vi "Teleop.vi"(10 "Match Info":T1={"Autonomous Elapsed Seconds"=0.0, "TeleOp Elapsed Seconds"=0.0, "Disabled Elapsed Seconds"=0.0, "Visited Autonomous"=FALSE, "Visited TeleOp"=FALSE, "Visited Disabled"=FALSE, "Autonomous Settings"={"Autonomous Style"=enum."Independent", "VI Refnum"=refnum}}, 11 "Call Context":T2) -> ()   [LabVIEW 2016]
doc: "This VI is called for each TeleOp packet received from the DS where the robot is not disabled. It is often used to read from the joysticks and update I/O or to update setpoints for timed control loops. It should complete and return within 20 milliseconds or it may miss DS packets."
uses:
  <vilib>/Rock Robotics/WPI/DriverStation/WPI_DriverStationDerivedRobotMode.ctl
  <vilib>/Rock Robotics/WPI/DriverStation/WPI_DriverStationMatch Info.ctl
  <vilib>/Rock Robotics/Network Tables/NT Read Boolean.vi
  <vilib>/Rock Robotics/Network Tables/NT Read Number.vi
  <vilib>/Rock Robotics/WPI/Utilities/WPI_GetSetVariantRefNum.vi
  <vilib>/Rock Robotics/Network Tables/NT Write Numeric Array.vi
  <vilib>/Rock Robotics/Network Tables/NT Write Boolean Array.vi
panel:
  out "Lift Bottom":dbl
  out "Lift Top":dbl
  out "Sample Slider 0":dbl(slide) scale=0.0..5.0
  out "Sample Boolean 1":bool
  out "Sample Boolean 0":bool
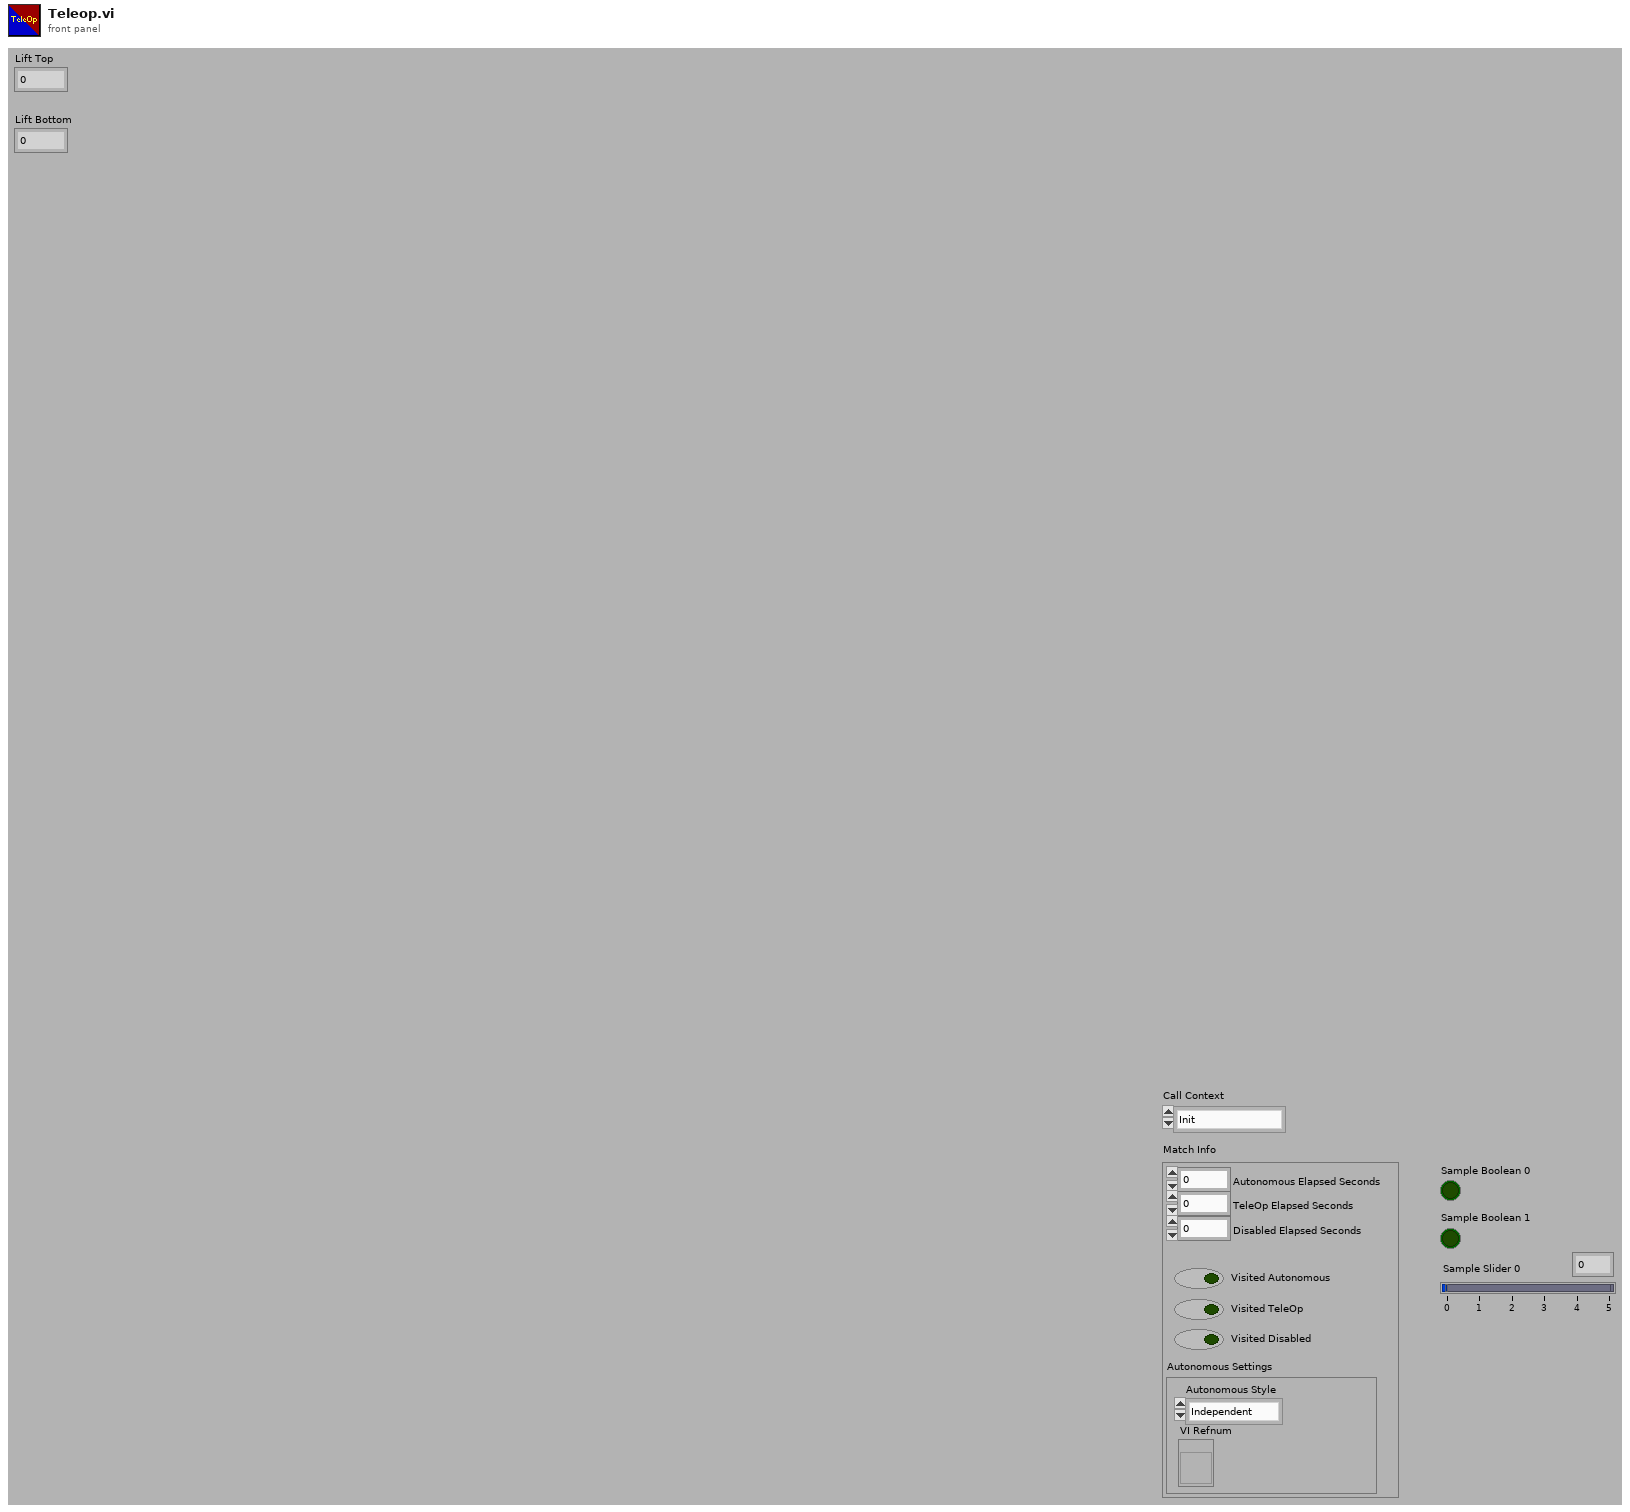
[diagram p1: front panel]
types:
  T1 = typedef "WPI_DriverStationMatch Info.ctl" = cluster{"Autonomous Elapsed Seconds":dbl, "TeleOp Elapsed Seconds":dbl, "Disabled Elapsed Seconds":dbl, "Visited Autonomous":bool, "Visited TeleOp":bool, "Visited Disabled":bool, "Autonomous Settings":cluster{"Autonomous Style":enum16{"Iterative", "Independent"}, "VI Refnum":refnum<vi>}}
  T2 = typedef "WPI_DriverStationDerivedRobotMode.ctl" = enum16{"Init", "Execute", "Stop"}
  T3 = typedef "WPI_JoystickDevRef.ctl" = cluster{"Device":T4}
  T4 = typedef "WPI_JoystickDeviceEnum.ctl" = enum16{"USB 0", "USB 1", "USB 2", "USB 3", "USB 4", "USB 5"}
  T5 = cluster{"Buttons[0]":bool, "Buttons[1]":bool, "Buttons[2]":bool, "Buttons[3]":bool, "Buttons[4]":bool, "Buttons[5]":bool, "Buttons[6]":bool, "Buttons[7]":bool, "Buttons[8]":bool}
  T6 = typedef "WPI_DigitalInputDevRef.ctl" = cluster{"DevStatus":errorcluster, "DIO Channel":T7}
  T7 = typedef "FPGA_DIOChannel.ctl" = enum8{"DIO 0", "DIO 1", "DIO 2", "DIO 3", "DIO 4", "DIO 5", "DIO 6", "DIO 7", "DIO 8", "DIO 9", "DIO MXP 0", "DIO MXP 1", "DIO MXP 2", "DIO MXP 3", "DIO MXP 4", "DIO MXP 5", "DIO MXP 6", "DIO MXP 7", "DIO MXP 8", "DIO MXP 9", "DIO MXP 10", "DIO MXP 11", "DIO MXP 12", "DIO MXP 13", "DIO MXP 14", "DIO MXP 15", "SPI Port CS1", "SPI Port CS2", "SPI Port CS3", "SPI Port MISO", "SPI Port MOSI", "Invalid"}
  T8 = typedef "WPI_RobotDriveDevRef.ctl" = cluster{"DevStatus":errorcluster, "Motors[]":T9[], "Square Inputs":bool, "Max Output":dbl}
  T9 = typedef "WPI_MotorControlDeviceRef.ctl" = cluster{"DeviceStatus":errorcluster, "Type":T10, "PWM":cluster{"PWM Channel":T11, "DeadBand":T12}, "CAN":cluster{"Device Number":u8, "SetOutput VI Ref":variant, "GetOutput VI Ref":variant, "Enable VI Ref":variant, "Disable VI Ref":variant, "Data":variant}, "Invert":bool}
  T10 = typedef "WPI_MotorControlType.ctl" = enum16{"PWM", "CAN"}
  T11 = typedef "FPGA_DIOPWMChannel.ctl" = enum8{"PWM 0", "PWM 1", "PWM 2", "PWM 3", "PWM 4", "PWM 5", "PWM 6", "PWM 7", "PWM 8", "PWM 9", "PWM MXP 0", "PWM MXP 1", "PWM MXP 2", "PWM MXP 3", "PWM MXP 4", "PWM MXP 5", "PWM MXP 6", "PWM MXP 7", "PWM MXP 8", "PWM MXP 9", "Invalid"}
  T12 = typedef "WPI_PWMDeadband.ctl" = cluster{"Name":string, "maxPositivePwm":i32, "minPositivePwm":i32, "centerPwm":i32, "maxNegativePwm":i32, "minNegativePwm":i32, "angularRange":u16}
  T13 = cluster{"Axes[0]":dbl, "Axes[1]":dbl, "Axes[2]":dbl, "Axes[3]":dbl, "Axes[4]":dbl, "Axes[5]":dbl, "Axes[6]":dbl, "Axes[7]":dbl, "Axes[8]":dbl}
  T14 = typedef "WPI_ServoDeviceRef.ctl" = cluster{"DeviceStatus":errorcluster, "PWM Channel":T11, "DeadBand":T12}
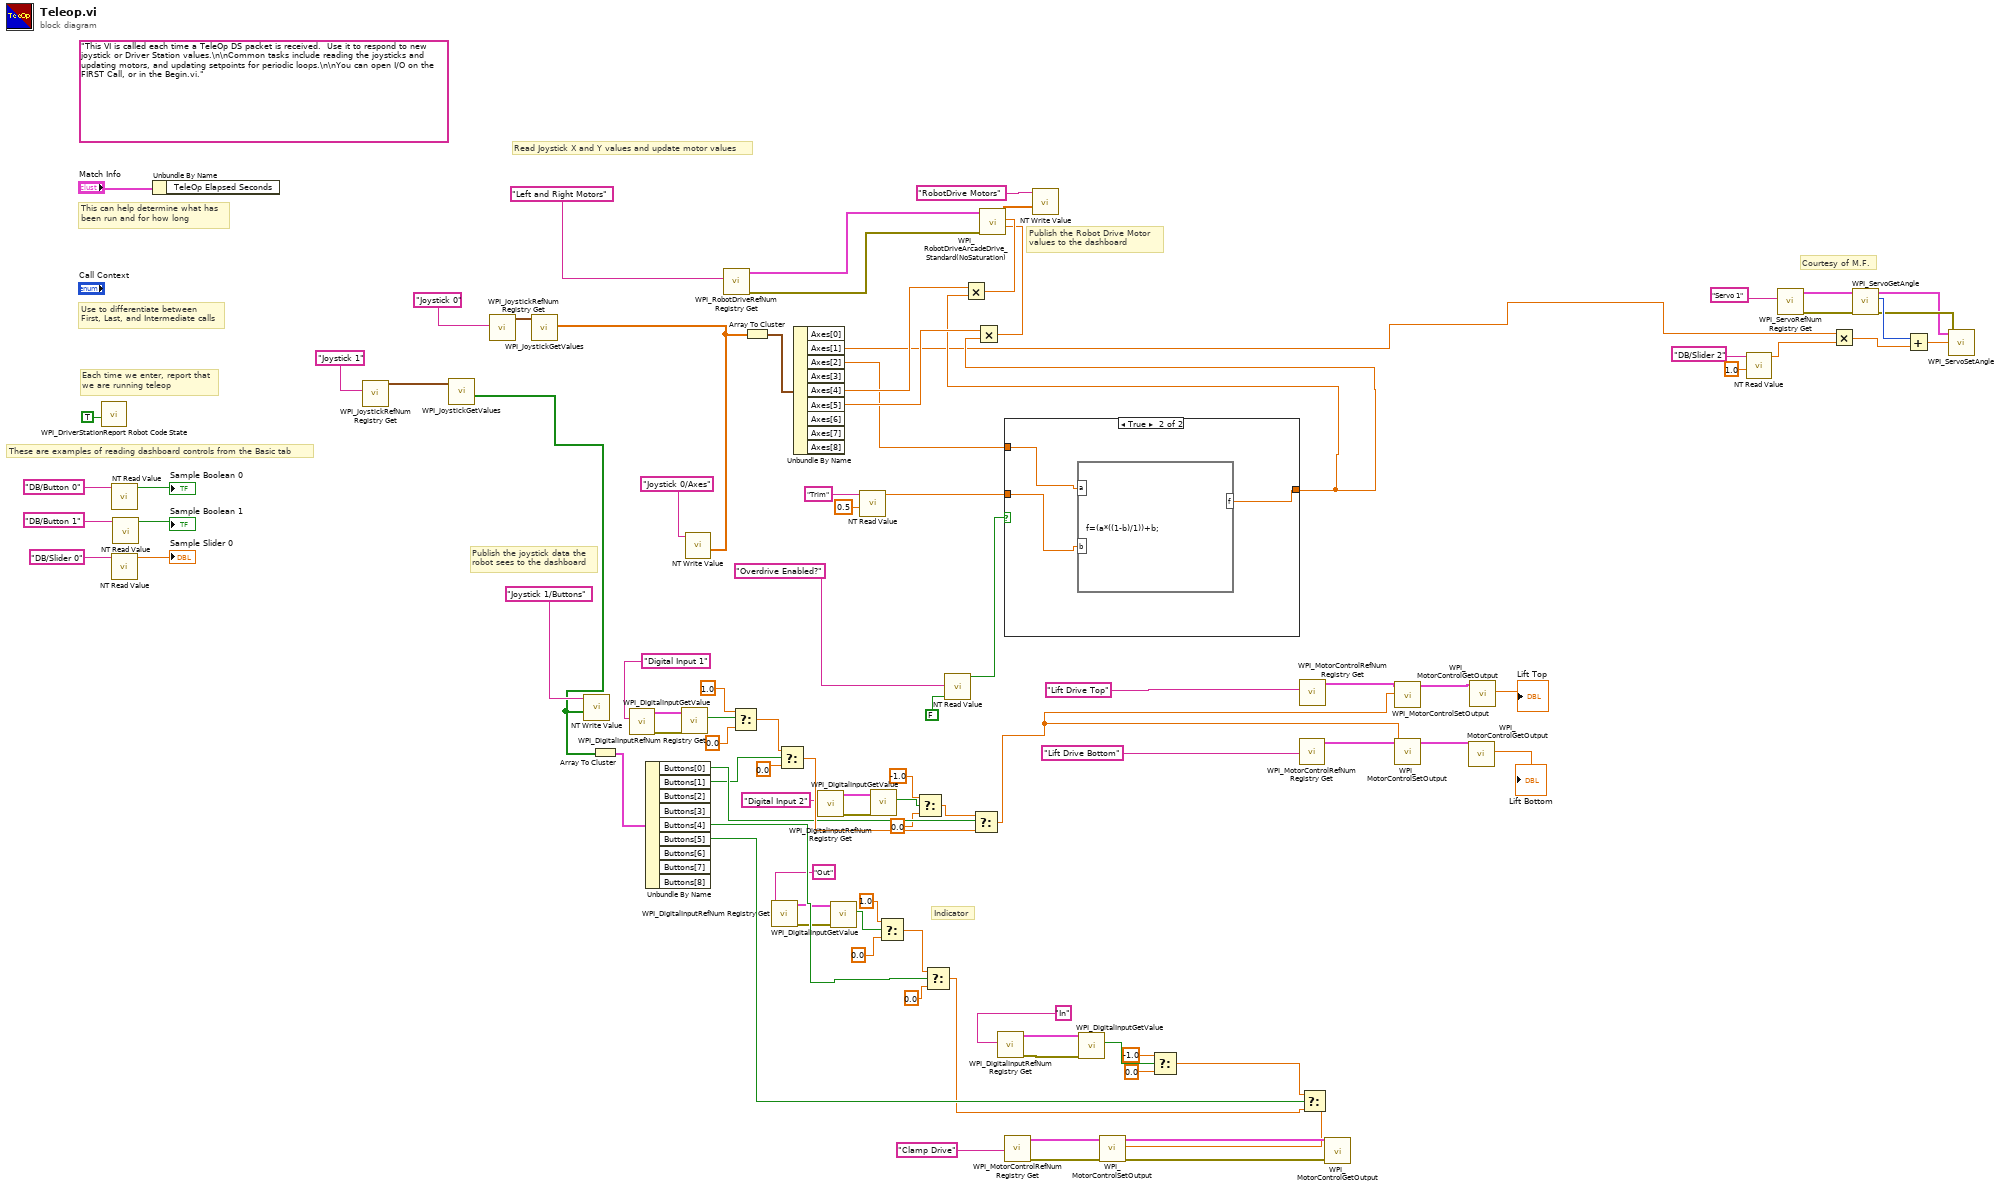
[diagram p0: block diagram]
diagram:
  (unwired) "This VI is called each time a TeleOp DS packet is received.  Use it to respond to new joystick or Driver Station values.\n\nCommon tasks include reading the joysticks and updating motors, and updating setpoints for periodic loops.\n\nYou can open I/O on the FIRST Call, or in the Begin.vi."
  # "Courtesy of M.F."
  # "Indicator"
  # "Publish the Robot Drive Motor\nvalues to the dashboard"
  # "Publish the joystick data the\nrobot sees to the dashboard"
  # "Read Joystick X and Y values and update motor values"
  # "These are examples of reading dashboard controls from the Basic tab"
  # "Each time we enter, report that\nwe are running teleop"
  # "Use to differentiate between\nFirst, Last, and Intermediate calls"
  # "This can help determine what has\nbeen run and for how long"
  n1 = call <vilib>:"WPI_DriverStationReport Robot Code State.vi"("TeleOp"=TRUE ("Autonomous")) -> ()  [unwired: 10 in, 1 out]
  n2 = call-poly <vilib>:"NT Read Value.vi"("Name"="DB/Button 0" ("refnum name")) -> ("Boolean"=→"Sample Boolean 0":bool)  [unwired: 9 in, 1 out]
  n3 = call-poly <vilib>:"NT Read Value.vi"("Name"="DB/Slider 0" ("refnum name")) -> ("Numeric"=→"Sample Slider 0":dbl)  [unwired: 9 in, 1 out]
  n4 = call-poly <vilib>:"NT Read Value.vi"("Name"="DB/Button 1" ("refnum name")) -> ("Boolean"=→"Sample Boolean 1":bool)  [unwired: 9 in, 1 out]
  n5 = Unbundle By Name("Match Info") -> ()  [unwired: 1 out]
  n6 = call <vilib>:"WPI_JoystickRefNum Registry Get.vi"("refnum name"="Joystick 1") -> ("JoystickDevRef"=w49:T3)  [unwired: 9 in, 1 out]
  n7 = call <vilib>:"WPI_JoystickGetValues.vi"("JoystickDevRef"=w49) -> ("Buttons"=w48:bool[])  [unwired: 6 in, 4 out]
  n8 = call <vilib>:"WPI_JoystickRefNum Registry Get.vi"("refnum name"="Joystick 0") -> ("JoystickDevRef"=w88:T3)  [unwired: 1 in, 9 out]
  n9 = call <vilib>:"WPI_JoystickGetValues.vi"("JoystickDevRef"=w88) -> ("Axes"=w63:dbl[])  [unwired: 6 in, 4 out]
  n10 = call-poly <vilib>:"NT Write Value.vi"("Boolean Array"=w48, "Name"="Joystick 1/Buttons") -> ()  [unwired: 9 in, 1 out]
  n11 = Array To Cluster(array=w48) -> (cluster=w64:T5)
  n12 = call <vilib>:"WPI_DigitalInputRefNum Registry Get.vi"("refnum name"="Digital Input 1") -> ("error out"=w30:errorcluster, "DigitalInputDevRef"=w31:T6)  [unwired: 9 in]
  n13 = Unbundle By Name(w64) -> ("Buttons[0]"=w50:bool, "Buttons[1]"=w27:bool, "Buttons[4]"=w24:bool, "Buttons[5]"=w26:bool)  [unwired: 5 out]
  n14 = call <vilib>:"WPI_DigitalInputGetValue.vi"("error in (no error)"=w30, "DigitalInputDevRef"=w31) -> ("Value"=w29:bool)  [unwired: 7 in, 2 out]
  n15 = call-poly <vilib>:"NT Write Value.vi"("Numeric Array"=w63, "Name"="Joystick 0/Axes") -> ()  [unwired: 9 in, 1 out]
  n16 = call <vilib>:"WPI_RobotDriveRefNum Registry Get.vi"("refnum name"="Left and Right Motors") -> ("error out"=w59:errorcluster, "RobotDriveDevRef"=w89:T8)  [unwired: 1 in, 8 out]
  n17 = Select(t=1.0, s=w29, f=0.0) -> (s? t:f=w40:dbl)
  n18 = Array To Cluster(array=w63) -> (cluster=w62:T13)
  n19 = call <vilib>:"WPI_DigitalInputRefNum Registry Get.vi"("refnum name"="Out") -> ("error out"=w14:errorcluster, "DigitalInputDevRef"=w23:T6)  [unwired: 9 in]
  n20 = Select(t=w40, s=w27, f=0.0) -> (s? t:f=w70:dbl)
  n21 = Unbundle By Name(w62) -> ("Axes[1]"=w2:dbl, "Axes[2]"=w51:dbl, "Axes[4]"=w61:dbl, "Axes[5]"=w60:dbl)  [unwired: 5 out]
  n22 = call <vilib>:"WPI_DigitalInputRefNum Registry Get.vi"("refnum name"="Digital Input 2") -> ("error out"=w34:errorcluster, "DigitalInputDevRef"=w35:T6)  [unwired: 9 in]
  n23 = call <vilib>:"WPI_DigitalInputGetValue.vi"("error in (no error)"=w14, "DigitalInputDevRef"=w23) -> ("Value"=w21:bool)  [unwired: 7 in, 2 out]
  n24 = call-poly <vilib>:"NT Read Value.vi"("Default Value"=0.5, "Name"="Trim" ("refnum name")) -> ("Numeric"=w55:dbl)  [unwired: 8 in, 1 out]
  n25 = call <vilib>:"WPI_DigitalInputGetValue.vi"("error in (no error)"=w34, "DigitalInputDevRef"=w35) -> ("Value"=w33:bool)  [unwired: 7 in, 2 out]
  n26 = Select(t=1.0, s=w21, f=0.0) -> (s? t:f=w18:dbl)
  n27 = Select(t=-1.0, s=w33, f=0.0) -> (s? t:f=w41:dbl)
  n28 = Select(t=w18, s=w24, f=0.0) -> (s? t:f=w15:dbl)
  n29 = call-poly <vilib>:"NT Read Value.vi"("Default Value"=FALSE, "Name"="Overdrive Enabled?" ("refnum name")) -> ("Boolean"=w57:bool)  [unwired: 8 in, 1 out]
  n30 = Select(t=w41, s=w50, f=w70) -> (s? t:f=w71:dbl)
  n31 = call <vilib>:"WPI_DigitalInputRefNum Registry Get.vi"("refnum name"="In") -> ("error out"=w45:errorcluster, "DigitalInputDevRef"=w47:T6)  [unwired: 9 in]
  n32 = case shown="True" w57 {
    tunnel: [w99 w100] -> w53
    tunnel: w55 -> [w99 w101]
    tunnel: w51 -> [_ w102]
    frame False {
    }
    frame True {
      n33 = formula code="f=(a*((1-b)/1))+b;"("a"=w102, "b"=w101) -> ("f"=w100:dbl)
    }
  }
  n34 = Multiply(x=w61, y=w53) -> (x*y=w81:dbl)
  n35 = Multiply(x=w60, y=w53) -> (x*y=w80:dbl)
  n36 = call <vilib>:"WPI_RobotDriveArcadeDrive_Standard(NoSaturation).vi"("error in (no error)"=w59, "Y axis value"=w80, "X axis value"=w81, "RobotDriveDevRef"=w89) -> ("Motor Values"=w84:dbl[])  [unwired: 7 out]
  n37 = call <vilib>:"WPI_MotorControlRefNum Registry Get.vi"("refnum name"="Clamp Drive") -> ("error out"=w69:errorcluster, "MotorControlDevRef"=w67:T9)  [unwired: 9 in]
  n38 = call-poly <vilib>:"NT Write Value.vi"("Numeric Array"=w84, "Name"="RobotDrive Motors") -> ()  [unwired: 9 in, 1 out]
  n39 = call <vilib>:"WPI_DigitalInputGetValue.vi"("error in (no error)"=w45, "DigitalInputDevRef"=w47) -> ("Value"=w43:bool)  [unwired: 7 in, 2 out]
  n40 = Select(t=-1.0, s=w43, f=0.0) -> (s? t:f=w16:dbl)
  n41 = call <vilib>:"WPI_MotorControlRefNum Registry Get.vi"("refnum name"="Lift Drive Bottom") -> ("MotorControlDevRef"=w76:T9)  [unwired: 9 in, 1 out]
  n42 = call <vilib>:"WPI_MotorControlRefNum Registry Get.vi"("refnum name"="Lift Drive Top") -> ("MotorControlDevRef"=w77:T9)  [unwired: 9 in, 1 out]
  n43 = Select(t=w16, s=w26, f=w15) -> (s? t:f=w42:dbl)
  n44 = call <vilib>:"WPI_MotorControlSetOutput.vi"("error in (no error)"=w69, "Output"=w42, "MotorControlDevRef"=w67) -> ("error out"=w66:errorcluster, "MotorControlDevRef"=w68:T9)  [unwired: 6 in, 1 out]
  n45 = call <vilib>:"WPI_MotorControlGetOutput.vi"("error in"=w66, "MotorControlDevRef"=w68) -> ()  [unwired: 7 in, 3 out]
  n46 = call <vilib>:"WPI_MotorControlSetOutput.vi"("Output"=w71, "MotorControlDevRef"=w77) -> ("MotorControlDevRef"=w78:T9)  [unwired: 7 in, 2 out]
  n47 = call <vilib>:"WPI_MotorControlSetOutput.vi"("Output"=w71, "MotorControlDevRef"=w76) -> ("MotorControlDevRef"=w79:T9)  [unwired: 7 in, 2 out]
  n48 = call <vilib>:"WPI_MotorControlGetOutput.vi"("MotorControlDevRef"=w79) -> ("Output"=→"Lift Bottom":dbl)  [unwired: 8 in, 2 out]
  n49 = call <vilib>:"WPI_MotorControlGetOutput.vi"("MotorControlDevRef"=w78) -> ("Output"=→"Lift Top":dbl)  [unwired: 8 in, 2 out]
  n50 = call-poly <vilib>:"NT Read Value.vi"("Default Value"=1.0, "Name"="DB/Slider 2" ("refnum name")) -> ("Numeric"=w8:dbl)  [unwired: 8 in, 1 out]
  n51 = call <vilib>:"WPI_ServoRefNum Registry Get.vi"("refnum name"="Servo 1") -> ("error out"=w5:errorcluster, "ServoDeviceRef"=w6:T14)  [unwired: 9 in]
  n52 = Multiply(x=w2, y=w8) -> (x*y=w11:dbl)
  n53 = call <vilib>:"WPI_ServoGetAngle.vi"("ServoDeviceRef"=w6, "error in (no error)"=w5) -> ("ServoDeviceRef"=w3:T14, "Angle"=w12:u16, "error out"=w4:errorcluster)  [unwired: 6 in]
  n54 = Add(x=w12, y=w11) -> (x+y=w13:dbl)
  n55 = call <vilib>:"WPI_ServoSetAngle.vi"("error in (no error)"=w4, "Angle"=w13, "ServoDeviceRef"=w3) -> ()  [unwired: 7 in, 2 out]
